vi "Init.vi"(8 "error in":errorcluster, 10 "PDO Communication Parameter Entry":refnum<class "OD Entry.lvclass">, 11 "Electronic Datasheet":refnum<class "Electronic Datasheet.lvclass">) -> (0 "error out":errorcluster, 3 "PDO Slot out":refnum<class "PDO Slot.lvclass">)   [LabVIEW 2019, in "PDO Grid.lvlib" / "PDO Slot.lvclass"]
uses:
  PDO Slot.lvclass
  PDO Slot.lvclass/PDO Slot.ctl
  RX PDO Mapping/RX PDO Mapping.lvclass
  TX PDO Mapping/TX PDO Mapping.lvclass
  RPDO Communication Parameter/RX PDO Communication Parameter.lvclass
  TPDO Communication Parameter/TX PDO Communication Parameter.lvclass
  Electronic Datasheet/Electronic Datasheet.lvclass
  Core/OD Entry/OD Entry.lvclass
  PDO Grid.lvlib
  PDO Mapping/PDO Mapping.lvclass
  Core/PDO Communication Parameter/PDO Communication Parameter.lvclass
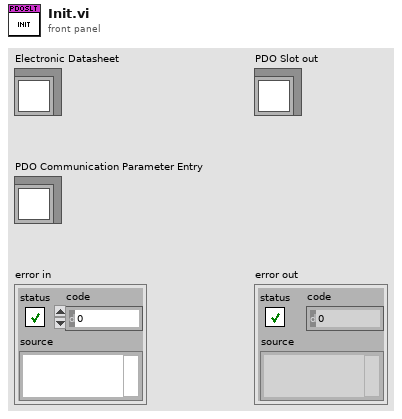
[diagram p1: front panel]
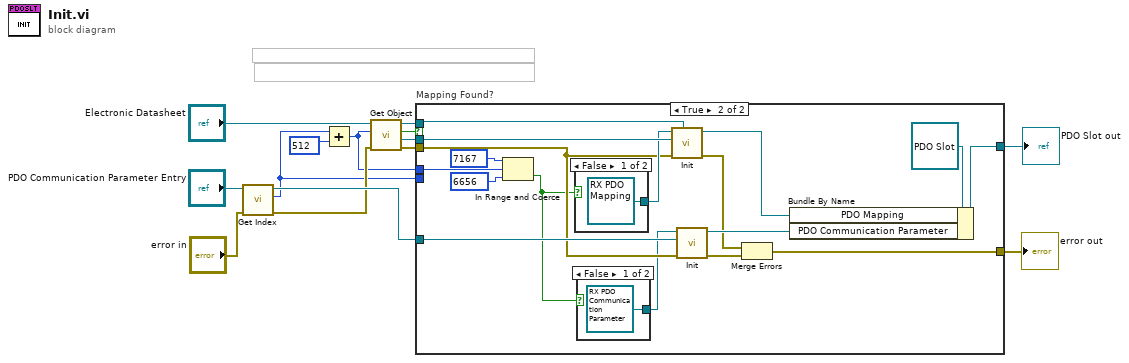
[diagram p0: block diagram]
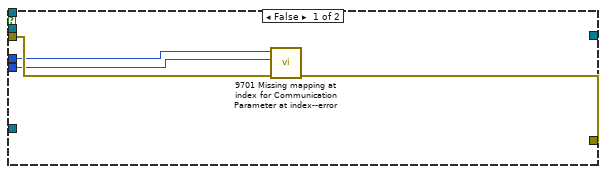
[diagram p2: hidden frame]
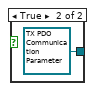
[diagram p3: hidden frame]
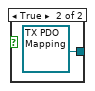
[diagram p4: hidden frame]
diagram:
  n1 = call "Get Index.vi"("Error In"="error in", "reference in"="PDO Communication Parameter Entry") -> ("Error Out"=w7:errorcluster, "Index"=w4:u16, "reference out"=w10:refnum<class "OD Entry.lvclass">)  [unwired: 7 in]
  n2 = Add(x=w4, y=u16 512) -> (x+y=w5:u16)
  n3 = call "Get Object.vi"("error in"=w7, "Index"=w5, "reference in"="Electronic Datasheet") -> ("error out"=w2:errorcluster, "OD Entry"=w1:refnum<class "OD Entry.lvclass">, "Found?"=w6:bool, "reference out"=w3:refnum<class "Electronic Datasheet.lvclass">)  [unwired: 5 in]
  n4 = case "Mapping Found?" shown="True" w6 {
    tunnel: [w17 w25] -> w14
    tunnel: [_ w33] -> w12
    tunnel: w10 -> [_ w31]
    tunnel: w2 -> [w18 w26]
    tunnel: w5 -> [w16 w23]
    tunnel: w4 -> [w15 _]
    tunnel: w3 -> [_ w29]
    tunnel: w1 -> [_ w30]
    frame False {
      n5 = call "9701 Missing mapping at index for Communication Parameter at index--error.vi"("error in"=w18, "Com Pam Index"=w15, "Mapping Index"=w16) -> ("error out"=w17:errorcluster)  [unwired: 8 in]
    }
    frame True {
      n6 = In Range and Coerce(upper limit=u16 7167, x=w23, lower limit=u16 6656 ("upper limit")) -> (In Range?=w20:bool)  [unwired: 1 out]
      n7 = case shown="False" w20 {
        tunnel: [refnum<class "RX PDO Mapping.lvclass"> refnum ("PDO Grid.lvlib:TPDO Mapping") refnum<class "TX PDO Mapping.lvclass"> refnum ("TPDO Mapping in")] -> w28
        frame False {
        }
        frame True {
        }
      }
      n8 = case shown="False" w20 {
        tunnel: [refnum<class "RX PDO Communication Parameter.lvclass"> refnum ("TPDO Mapping in") refnum<class "TX PDO Communication Parameter.lvclass"> refnum ("PDO Grid.lvlib:TX PDO Communication Parameter.lvclass")] -> w19
        frame False {
        }
        frame True {
        }
      }
      n9 = call-dynamic "Init.vi"("EDS"=w29, "error in"=w26, "OD Entry"=w30, "PDO Mapping in"=w28) -> ("error out"=w24:errorcluster, "PDO Mapping out"=w27:refnum<class "PDO Mapping.lvclass">)  [unwired: 6 in]
      n10 = call-dynamic "Init.vi"("error in"=w26, "OD Entry"=w31, "PDO Communication Parameter in"=w19) -> ("error out"=w35:errorcluster, "PDO Communication Parameter out"=w32:refnum<class "PDO Communication Parameter.lvclass">)  [unwired: 7 in]
      n11 = Merge Errors(w24, w35) -> (w25:errorcluster)
      n12 = Bundle By Name(cluster=refnum<class "PDO Slot.lvclass"> refnum ("PDO Slot out"), "PDO Mapping"=w27, "PDO Communication Parameter"=w32) -> (w33:refnum<class "PDO Slot.lvclass">)
    }
  }
  "error out" <- w14
  "PDO Slot out" <- w12
